vi "APEX_Measured_Spectrum_Examples.vi"(0 "APEX_VISA_IN":refnum<visa-resource-name>="APEX_OSA", 1 "Center(nm or GHz)":dbl=1550.0, 2 "Span (nm or GHz)":dbl=5.0, 3 "Freq_or_Wavelength":enum16{"Wavelength", "Frequency"}(ring), 7 "Resolution(MHz)":enum16{"5MHz", "140MHz", "2000MHz", "4000MHz"}(ring), 9 "Resolution(pm)":enum16{"0.04pm", "1.12pm", "10pm", "20pm"}(ring), 11 "error in":errorcluster, 13 "Trace number (1-6)":i8=1, 14 "Points number":i32=2000) -> (6 "XY Graph":cluster{dbl[], dbl[]}(graph), 15 "error out":errorcluster)   [LabVIEW 2020]
panel:
  out "X_Axis":dbl[](array[numeric]) format="%#_9g"
  out "read buffer 2":string
  out "return count 2":u32
  out "Power":dbl[](array[numeric])
  out "read buffer":string
  out "return count":u32
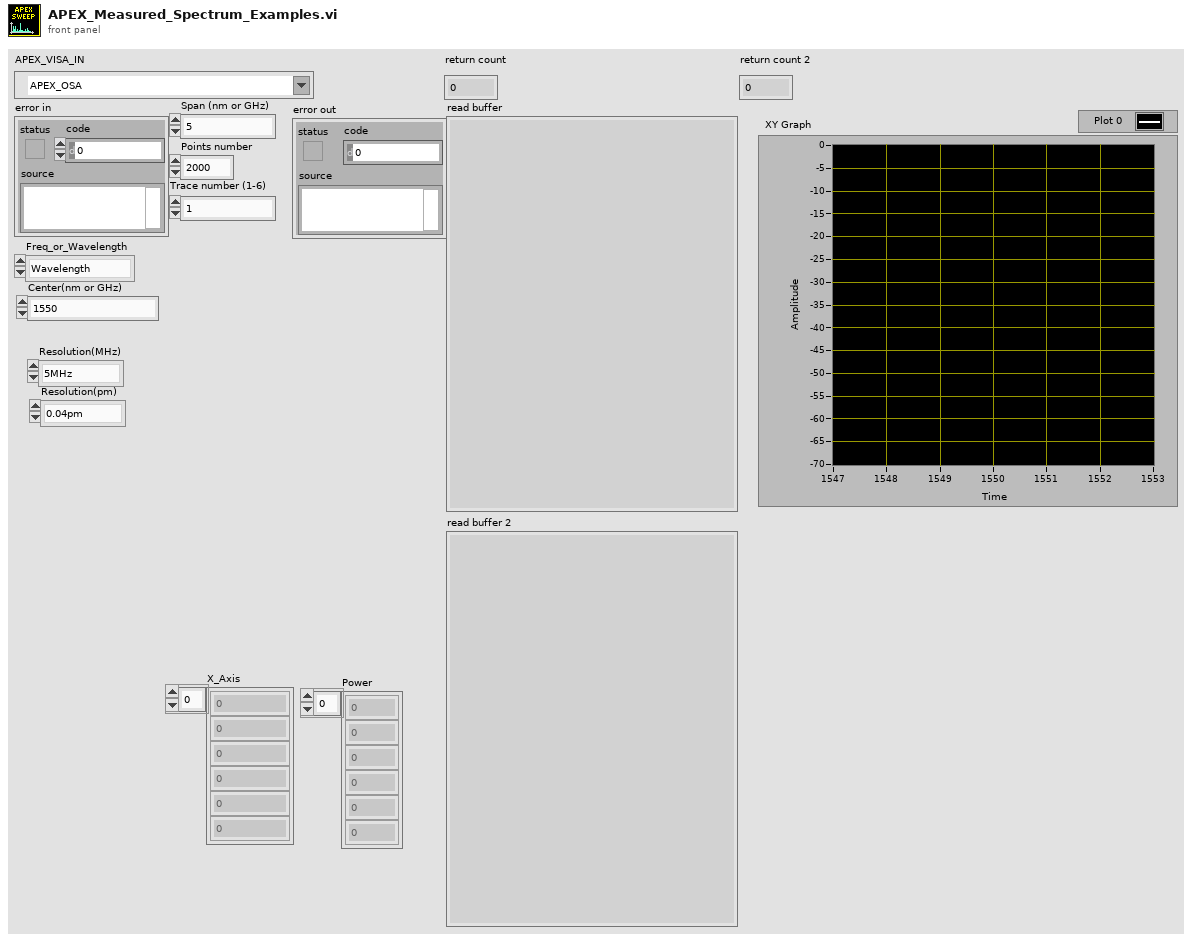
[diagram p1: front panel]
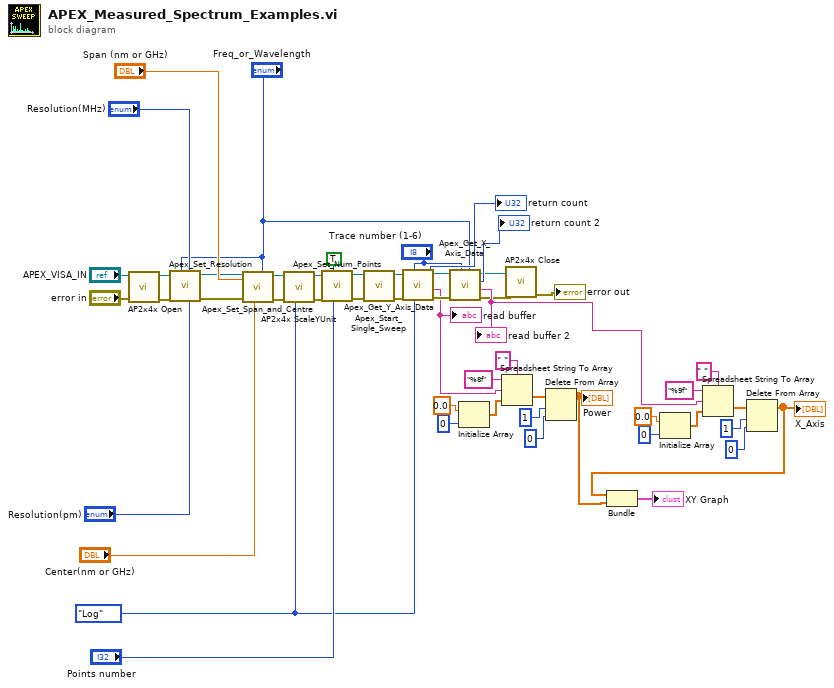
[diagram p0: block diagram]
diagram:
  w37 = enum16{"Linear", "Log"}."Log" ("Unit")
  n1 = call "AP2x4x Open.vi"("error in (no error)"="error in", "AP2x4x IN"="APEX_VISA_IN") -> ("error out"=w4:errorcluster, "AP2x4x OUT"=w5:refnum<visa-resource-name>)  [unwired: 8 in]
  n2 = call "Apex_Set_Resolution.vi"("Resolution(pm)"="Resolution(pm)", "Resolution(MHz)"="Resolution(MHz)", "Freq_or_Wavelength"="Freq_or_Wavelength", "error in"=w4, "APEX_VISA_IN"=w5) -> ("error out"=w2:errorcluster, "Apex_Out"=w3:refnum<visa-resource-name>)  [unwired: 5 in]
  n3 = call "Apex_Set_Span_and_Centre.vi"("Freq_or_Wavelength"="Freq_or_Wavelength", "Center(nm or GHz)"="Center(nm or GHz)", "Span (nm or GHz)"="Span (nm or GHz)", "error in"=w2, "AP2x4x IN"=w3) -> ("error out"=w42:errorcluster, "AP2x4x OUT"=w43:refnum<visa-resource-name>)  [unwired: 5 in]
  n4 = call "AP2x4x ScaleYUnit.vi"("Unit"=w37, "error in"=w42, "AP2x4x IN"=w43) -> ("error out"=w40:errorcluster, "AP2x4x OUT"=w41:refnum<visa-resource-name>)  [unwired: 7 in]
  n5 = call "Apex_Set_Num_Points.vi"("Points number"="Points number", "T = manual, F = auto"=TRUE, "error in"=w40, "AP2x4x IN"=w41) -> ("error out"=w47:errorcluster, "AP2x4x OUT"=w46:refnum<visa-resource-name>)  [unwired: 6 in]
  n6 = call "Apex_Start_Single_Sweep.vi"("error in"=w47, "AP2x4x IN"=w46) -> ("error out"=w39:errorcluster, "AP2x4x OUT"=w38:refnum<visa-resource-name>)  [unwired: 8 in]
  n7 = call "Apex_Get_Y_Axis_Data.vi"("Data scale"=w37, "Trace number (1-6)"="Trace number (1-6)", "error in"=w39, "AP2x4x IN"=w38) -> ("error out"=w26:errorcluster, "read buffer"=w23:string, "return count"=→"return count":u32, "AP2x4x OUT"=w27:refnum<visa-resource-name>)  [unwired: 3 in]
  "read buffer" <- w23
  n8 = call "Apex_Get_X_Axis_Data.vi"("Freq_or_Wavelength"="Freq_or_Wavelength", "Trace number (1-6)"="Trace number (1-6)", "error in"=w26, "AP2x4x IN"=w27) -> ("error out"=w13:errorcluster, "read buffer"=w15:string, "return count"=→"return count 2":u32, "AP2x4x OUT"=w14:refnum<visa-resource-name>)  [unwired: 3 in]
  "read buffer 2" <- w15
  n9 = Initialize Array(0.0 ("element"), 0 ("dimension size")) -> (w35:dbl[])
  n10 = Spreadsheet String To Array(delimiter (Tab)=" ", format string="%8f", spreadsheet string=w23, array type (2D Dbl)=w35) -> (array=w28:dbl[])
  n11 = call "AP2x4x Close.vi"("error in (no error)"=w13, "AP2x4x IN"=w14) -> ("error out"=→"error out":errorcluster)  [unwired: 9 in]
  n12 = Delete From Array(array=w28, length=1, index=0) -> (array with subset deleted=w11:dbl[])  [unwired: 1 out]
  "Power" <- w11
  n13 = Initialize Array(0.0 ("element"), 0 ("dimension size")) -> (w16:dbl[])
  n14 = Spreadsheet String To Array(delimiter (Tab)=" ", format string="%9f", spreadsheet string=w15, array type (2D Dbl)=w16) -> (array=w9:dbl[])
  n15 = Delete From Array(array=w9, length=1, index=0) -> (array with subset deleted=w8:dbl[])  [unwired: 1 out]
  "X_Axis" <- w8
  n16 = Bundle(w8, w11) -> (→"XY Graph":cluster{dbl[], dbl[]})  [unwired: 1 in]
